vi "StreamWebSocket.vi"(8 "error in":errorcluster) -> (0 "error out":errorcluster)   [LabVIEW 2024]
uses:
  GlobalVars/webSocketVars.vi
  <vilib>/MediaMongrels Ltd/WebSockets/WebSockets/WebSocket Server/WebSocket Server.lvclass
panel:
  out "Array":string[](array[string])
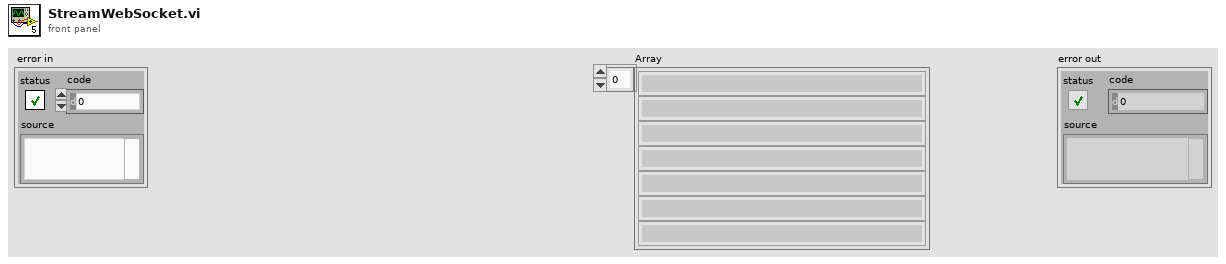
[diagram p1: front panel]
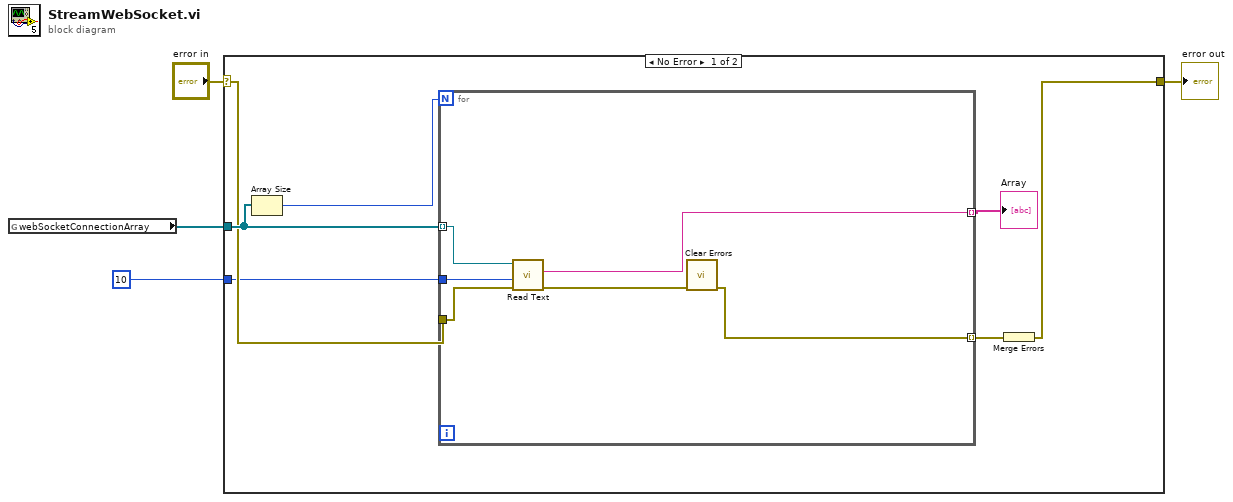
[diagram p0: block diagram]
diagram:
  n1 = global read "webSocketVars.vi" "webSocketConnectionArray"() -> (w2:refnum<class "WebSocket Server.lvclass">[])
  n2 = case shown="No Error" "error in" {
    selector: "error in" -> [w9 w18]
    tunnel: [w6 w18] -> w3
    tunnel: w2 -> [w11 _]
    tunnel: 10 ("timeout ms (5000)") -> [w8 _]
    frame No Error {
      n3 = Array Size(array=w11) -> (size(s)=w10:i32)
      n4 = for {
        N: w10 -> [_]
        tunnel: w11 -> [w17] mode=indexing
        tunnel: w9 -> [w15]
        tunnel: w8 -> [w16]
        tunnel: [w13] -> w7 mode=indexing
        tunnel: [w12] -> w5 mode=indexing
        n5 = call-dynamic "Read Text.vi"("error in (no error)"=w15, "timeout ms (5000)"=w16, "WebSocket in"=w17) -> ("error out"=w14:errorcluster, "Data"=w12:string)  [unwired: 6 in, 1 out]
        n6 = call <vilib>:"Clear Errors.vi"("error in (no error)"=w14) -> ("error out"=w13:errorcluster)  [unwired: 5 in, 1 out]
      }
      "Array" <- w5
      n7 = Merge Errors(w7) -> (w6:errorcluster)
    }
    frame Error {
    }
  }
  "error out" <- w3
